vi "PH_Beckhoff_PP_Control.declare analog InputTags.vi"() -> (0 "Analog Inputs":T3, 1 "Description":string)   [LabVIEW 2014, in "PH_Beckhoff_PP_Control.lvlib"]
uses:
  PH_Beckhoff_PP_Control.lvlib
  PH_Beckhoff/PH_Beckhoff.Analog Inputs.ctl
  PH_Beckhoff/PH_Beckhoff.Scaling Type.ctl
  PH_Beckhoff_PP_Control.PP Mercury Tags.ctl
  PH_Beckhoff_PP_Control.PP Conductivity Tags.ctl
  PH_Beckhoff/PH_Beckhoff.lvlib
panel:
  in  "Analog Input Value":T2
  out "Right Size?":bool
  # "Let this VI run to check the size!"
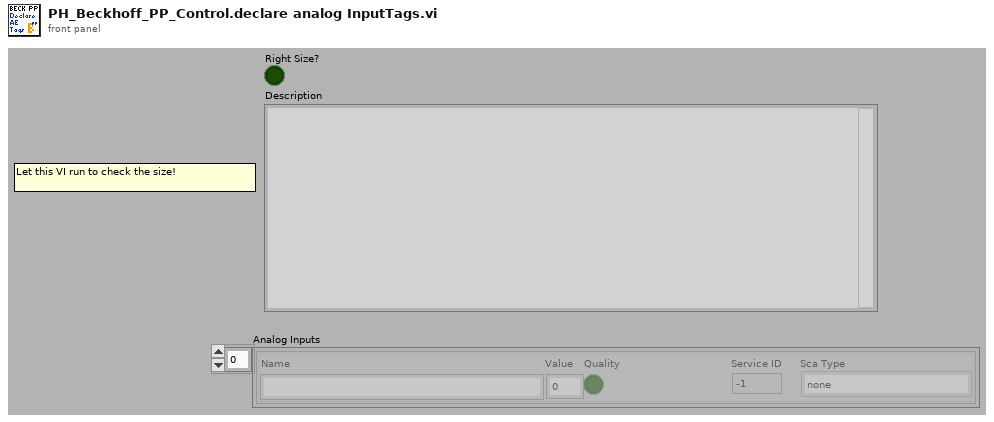
[diagram p1: front panel]
types:
  T1 = typedef "PH_Beckhoff.lvlib/PH_Beckhoff.Scaling Type.ctl" = enum16{"none", "0 ... 15 Bit -> 0 ... 5", "0 ... 15 Bit -> 0 ... 10", "0 ... 15 Bit -> 0 ... 25", "0 ... 15 Bit -> 4 ... 20", "0 ... 15 Bit -> 0 ... 1", "0 ... 15 Bit -> 0 ... 20000", "0 ... 15 Bit -> 0 ... 24000"}
  T2 = cluster{"Name":string, "Value":u32, "Quality":bool, "Service ID":i32, "Sca Type":T1}
  T3 = typedef "PH_Beckhoff.lvlib/PH_Beckhoff.Analog Inputs.ctl" = cluster{"Name":string, "Value":u32, "Quality":bool, "Service ID":i32, "Sca Type":T1}[]
  T4 = typedef "PH_Beckhoff_PP_Control.lvlib/PH_Beckhoff_PP_Control.PP Conductivity Tags.ctl" = enum16{"Device-on", "Conductivity-2-high", "Temperature-not-2-low", "Alarm", "Conductivity", "Status"}
  T5 = typedef "PH_Beckhoff_PP_Control.lvlib/PH_Beckhoff_PP_Control.PP Mercury Tags.ctl" = enum16{"Device-on", "Alarm", "on-since", "Concentration", "Status"}
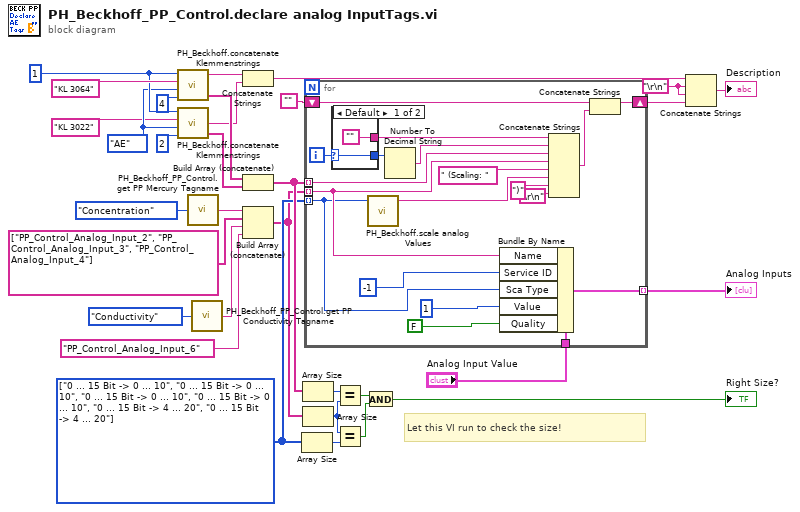
[diagram p0: block diagram]
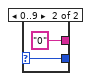
[diagram p2: hidden frame]
diagram:
  w9 = T1[] [enum."0 ... 15 Bit -> 0 ... 10", enum."0 ... 15 Bit -> 0 ... 10", enum."0 ... 15 Bit -> 0 ... 10", enum."0 ... 15 Bit -> 0 ... 10", enum."0 ... 15 Bit -> 4 ... 20", enum."0 ... 15 Bit -> 4 ... 20"] items=["none", "0 ... 15 Bit -> 0 ... 5", "0 ... 15 Bit -> 0 ... 10", "0 ... 15 Bit -> 0 ... 25", "0 ... 15 Bit -> 4 ... 20", "0 ... 15 Bit -> 0 ... 1", "0 ... 15 Bit -> 0 ... 20000", "0 ... 15 Bit -> 0 ... 24000"]
  w20 = 1 ("Quantity")
  w30 = "\r\n"
  w19 = enum16{"AE", "AA", "DE", "DA"}."AE" ("Type")
  # "Let this VI run to check the size!"
  n1 = call "PH_Beckhoff.concatenate Klemmenstrings.vi"("# of In- or Outputs"=4, "Type"=w19, "Klemmenname"="KL 3064", "Quantity"=w20) -> ("concatenated string array"=w14:string[], "\"<Type>: <Quantity> x <Klemmenname>\""=w11:string)  [unwired: 1 out]
  n2 = call "PH_Beckhoff.concatenate Klemmenstrings.vi"("# of In- or Outputs"=2, "Type"=w19, "Klemmenname"="KL 3022", "Quantity"=w20) -> ("concatenated string array"=w15:string[], "\"and <Quantity> x <Klemmenname>\""=w12:string)  [unwired: 1 out]
  n3 = call "PH_Beckhoff_PP_Control.get PP Mercury Tagname.vi"("PP Mercury Tag"=PH_Beckhoff_PP_Control.PP_Mercury_Tags."Concentration") -> ("PP Mercury Tagname"=w5:string)
  n4 = call "PH_Beckhoff_PP_Control.get PP Conductivity Tagname.vi"("PP Conductivity Tag"=PH_Beckhoff_PP_Control.PP_Conductivity_Tags."Conductivity") -> ("PP Conductivity Tagname"=w3:string)
  n5 = Concatenate Strings(w11, w12) -> (w16:string)
  n6 = Build Array (concatenate)(w14, w15) -> (w13:string[])
  n7 = Build Array (concatenate)(w5, string[] ["PP_Control_Analog_Input_2", "PP_Control_Analog_Input_3", "PP_Control_Analog_Input_4"], w3, "PP_Control_Analog_Input_6") -> (w1:string[])
  n8 = Array Size(array=w9) -> (size(s)=w23:i32)
  n9 = Array Size(array=w13) -> (size(s)=w28:i32)
  n10 = Array Size(array=w1) -> (size(s)=w24:i32)
  n11 = for {
    tunnel: w1 -> [w39] mode=indexing
    tunnel: w13 -> [w47] mode=indexing
    shift-right: [w44] -> w31
    shift-left: "" -> [w43]
    tunnel: w9 -> [w34] mode=indexing
    tunnel: "Analog Input Value" -> [w37]
    tunnel: [w33] -> w10 mode=indexing
    i -> [w51]
    n12 = case shown="Default" w51 {
      selector: w51 -> [w52 w55]
      tunnel: [w52 w55] -> w50
      tunnel: ["" "0"] -> w49
      frame Default {
      }
      frame 0..9 {
      }
    }
    n13 = call "PH_Beckhoff.scale analog Values.vi"("Sca Type"=w34) -> ("Scaling"=w42:string)  [unwired: 2 in, 2 out]
    n14 = Number To Decimal String(number=w50) -> (decimal integer string=w48:string)  [unwired: 1 in]
    n15 = Bundle By Name(cluster=w37, "Name"=w39, "Service ID"=-1, "Sca Type"=w34, "Value"=u32 1, "Quality"=FALSE) -> (w33:T2)
    n16 = Concatenate Strings(w49, w48, w47, w39, " (Scaling: " ("string"), w42, ")" ("string"), "\r\n") -> (w45:string)
    n17 = Concatenate Strings(w43, w45) -> (w44:string)
  }
  "Analog Inputs" <- w10
  n18 = Equal?(x=w28, y=w24) -> (x = y?=w27:bool)
  n19 = Equal?(x=w24, y=w23) -> (x = y?=w21:bool)
  n20 = And(x=w27, y=w21) -> (x .and. y?=→"Right Size?":bool)
  n21 = Concatenate Strings(w16, w30, w30, w31) -> (→"Description":string)
